vi "Threshold detection VI.vi"(11 "Windowed Frames":dbl[][](array[numeric])) -> (1 "Threshold Energy":dbl, 2 "Energy Graph":dbl[](graph), 3 "Boolean frame energy":i16[](array[numeric]))   [LabVIEW 2013]
uses:
  <vilib>/Analysis/baseanly.llb/Mean (DBL).vi
  <vilib>/Analysis/NI_AALBase.lvlib
panel:
  out "sum":dbl
  out "size(s)":i32
  out "Array - Numeric":dbl[](array[numeric])
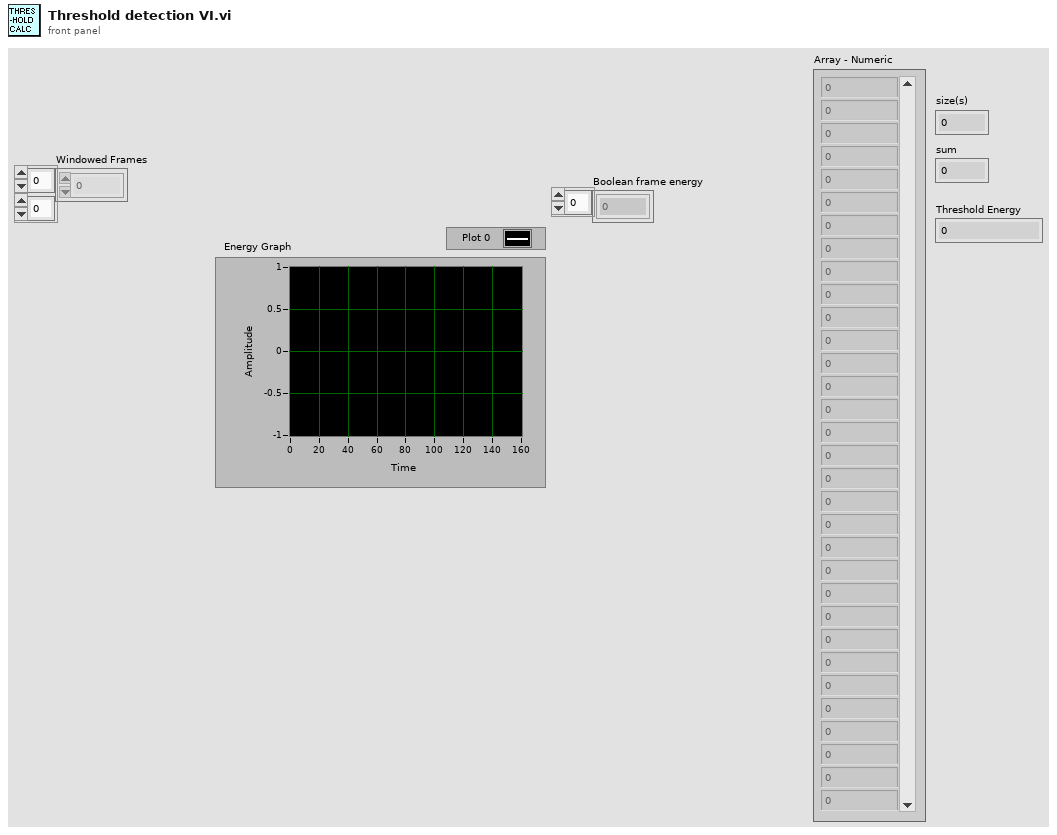
[diagram p1: front panel]
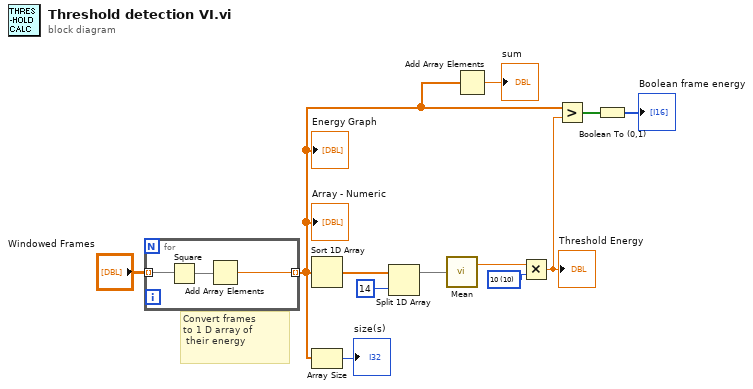
[diagram p0: block diagram]
diagram:
  w11 = u16 10 items=["5"=5, "6"=6, "7"=7, "9"=9, "10"=10]
  # "Convert frames \nto 1 D array of\n their energy"
  n1 = for {
    tunnel: "Windowed Frames" -> [w15] mode=indexing
    tunnel: [w13] -> w2 mode=indexing
    n2 = Square(x=w15) -> (x^2=w14:dbl[])
    n3 = Add Array Elements(numeric array=w14) -> (sum=w13:dbl)
  }
  "Energy Graph" <- w2
  "Array - Numeric" <- w2
  n4 = Sort 1D Array(array=w2) -> (sorted array=w6:dbl[])
  n5 = Array Size(array=w2) -> (size(s)=→"size(s)":i32)
  n6 = Split 1D Array(array=w6, index=14) -> (first subarray=w4:dbl[])  [unwired: 1 out]
  n7 = call-poly <vilib>:"Mean.vi"("X"=w4) -> ("mean"=w3:dbl)  [unwired: 1 out]
  n8 = Add Array Elements(numeric array=w2) -> (sum=→"sum":dbl)
  n9 = Multiply(x=w3, y=w11) -> (x*y=w10:dbl)
  "Threshold Energy" <- w10
  n10 = Greater?(x=w2, y=w10) -> (0:w9:bool[])
  n11 = Boolean To (0,1)(Boolean=w9) -> (0, 1=→"Boolean frame energy":i16[])
